vi "switchOff.vi"(8 "error in (no error)":errorcluster, 11 "AndorIKonTempController in":refnum<class "AndorIKonTempController.lvclass">) -> (0 "error out":errorcluster, 3 "AndorIKonTempController out":refnum<class "AndorIKonTempController.lvclass">)   [LabVIEW 2009, in "Hardware.lvlib" / "Channels.lvlib" / "AndorIKonTempController.lvclass"]
uses:
  AndorIKonTempController.lvclass
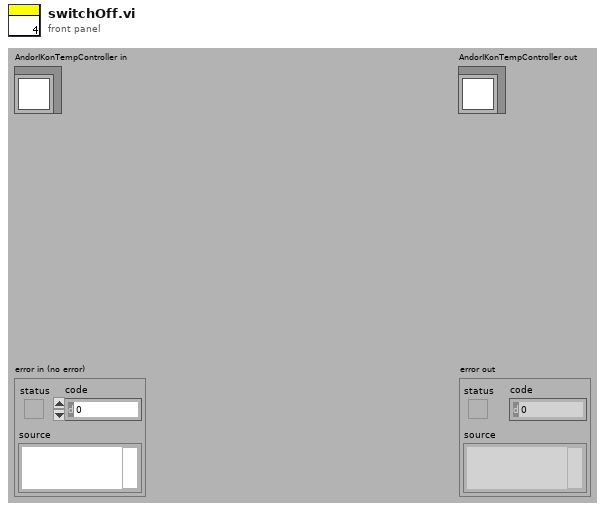
[diagram p1: front panel]
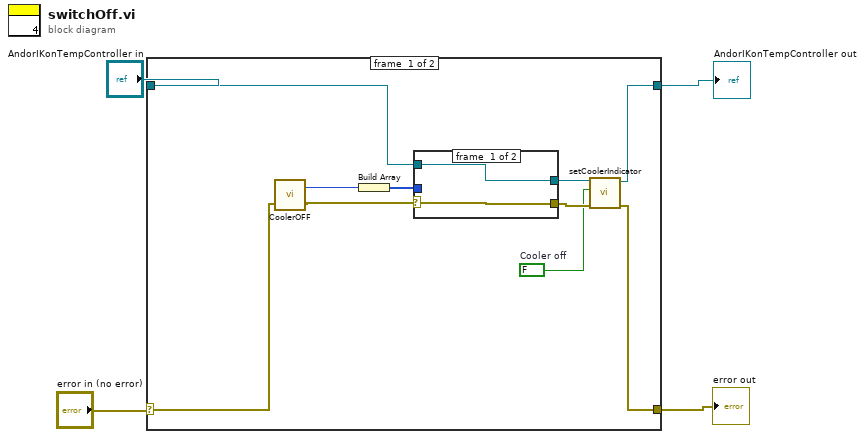
[diagram p0: block diagram]
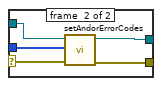
[diagram p2: hidden frame]
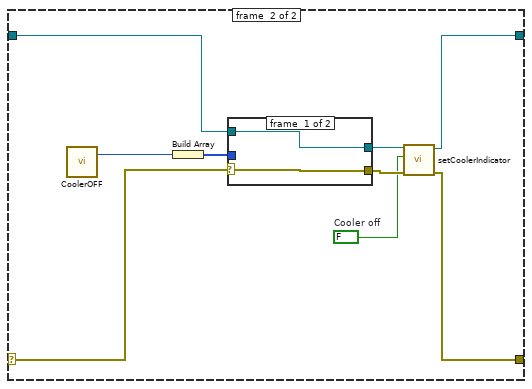
[diagram p3: hidden frame]
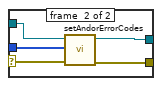
[diagram p4: hidden frame]
diagram:
  n1 = case shown="Error" "error in (no error)" {
    selector: "error in (no error)" -> [w11 w24]
    tunnel: [w6 w23] -> w2
    tunnel: "AndorIKonTempController in" -> [w10 w25]
    tunnel: [w5 w22] -> w1
    frame #0 {
      w7 = FALSE  # Cooler off
      n2 = call <userlib>:"CoolerOFF.vi"("error in (no error)"=w11) -> ("error out"=w13:errorcluster, "DLL error code"=w12:u32)  [unwired: 1 in]
      n3 = Build Array(w12) -> (w14:u32[])
      n4 = case shown="Error" w13 {
        selector: w13 -> [w16 w19]
        tunnel: [w16 w18] -> w8
        tunnel: w14 -> [_ w21]
        tunnel: w10 -> [w15 w20]
        tunnel: [w15 w17] -> w9
        frame #0 {
        }
        frame #1 {
          n5 = call-dynamic "setAndorErrorCodes.vi"("error in (no error)"=w19, "Andor Error Codes"=w21, "AndorIKonTempController.lvclass in"=w20) -> ("error out"=w18:errorcluster, "AndorIKonTempController.lvclass out"=w17:refnum<class "AndorIKonTempController.lvclass">)  [unwired: 7 in]
        }
      }
      n6 = call-dynamic "setCoolerIndicator.vi"("error in (no error)"=w8, "Cooler"=w7, "CameraTempController.lvclass in"=w9) -> ("error out"=w5:errorcluster, "CameraTempController.lvclass out"=w6:refnum<class "AndorIKonTempController.lvclass">)  [unwired: 7 in]
    }
    frame #1 {
      w26 = FALSE  # Cooler off
      n7 = call <userlib>:"CoolerOFF.vi"() -> ("DLL error code"=w29:u32)  [unwired: 2 in, 1 out]
      n8 = Build Array(w29) -> (w30:u32[])
      n9 = case shown="Error" w24 {
        selector: w24 -> [w32 w35]
        tunnel: [w32 w34] -> w27
        tunnel: w30 -> [_ w37]
        tunnel: w25 -> [w31 w36]
        tunnel: [w31 w33] -> w28
        frame #0 {
        }
        frame #1 {
          n10 = call-dynamic "setAndorErrorCodes.vi"("error in (no error)"=w35, "Andor Error Codes"=w37, "AndorIKonTempController.lvclass in"=w36) -> ("error out"=w34:errorcluster, "AndorIKonTempController.lvclass out"=w33:refnum<class "AndorIKonTempController.lvclass">)  [unwired: 7 in]
        }
      }
      n11 = call-dynamic "setCoolerIndicator.vi"("error in (no error)"=w27, "Cooler"=w26, "CameraTempController.lvclass in"=w28) -> ("error out"=w22:errorcluster, "CameraTempController.lvclass out"=w23:refnum<class "AndorIKonTempController.lvclass">)  [unwired: 7 in]
    }
  }
  "error out" <- w1
  "AndorIKonTempController out" <- w2
